vi "S19 Read.vi"(8 "error in":errorcluster, 11 "Flash File Path":path=path "D:/Gex 2 Flash Tool/SW_1_9_7_CT_0_4_2.s19") -> (0 "error out":errorcluster, 3 "Messages":T1[](array[typedef]) {"address" format="%x"; "Byte Array" format="%.0x"})   [LabVIEW 2018]
uses:
  type defs/s messages.ctl
panel:
  in  "message length (nibbles)":i32=512
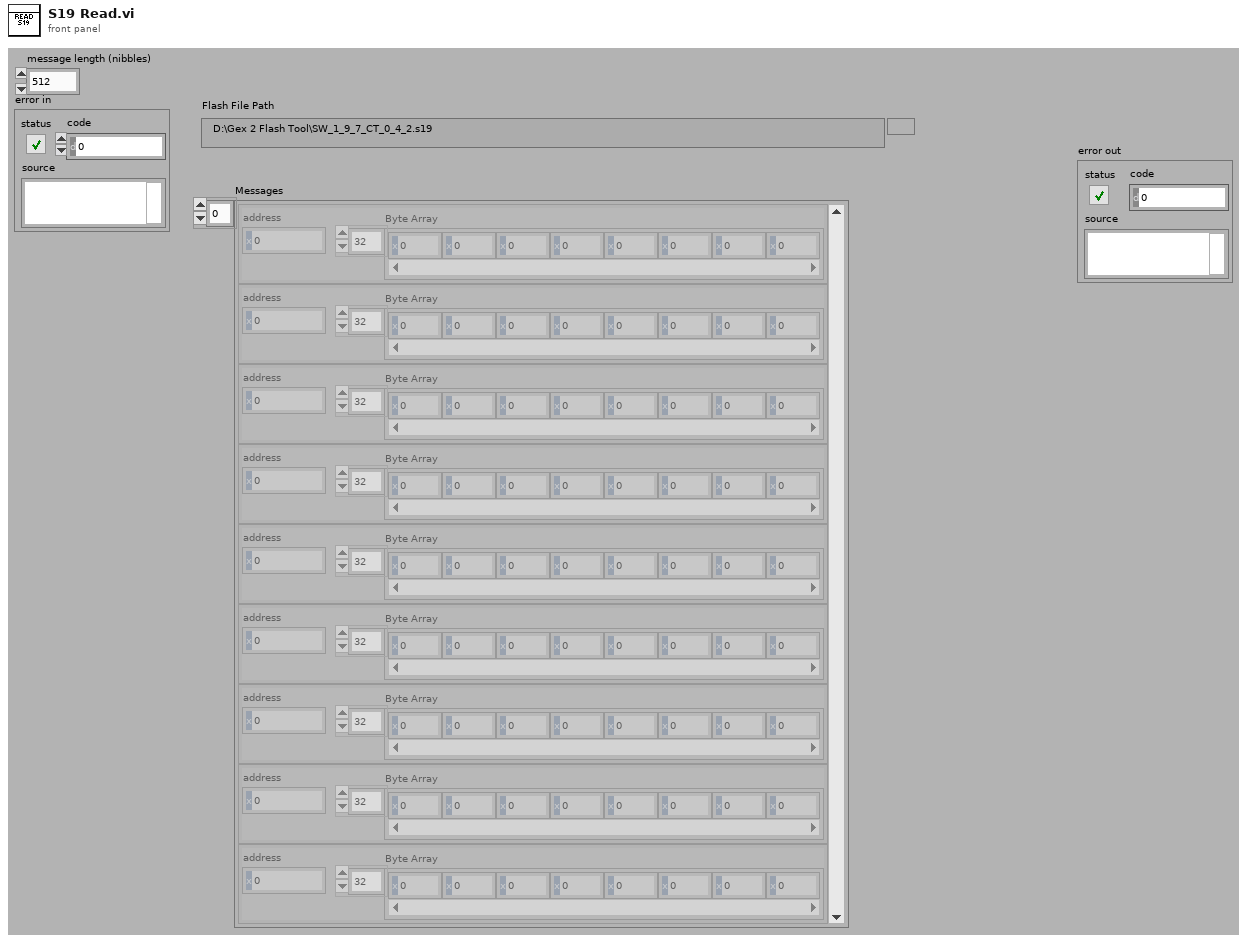
[diagram p1: front panel]
types:
  T1 = typedef "s messages.ctl" = cluster{"address":u32, "Byte Array":u8[]}
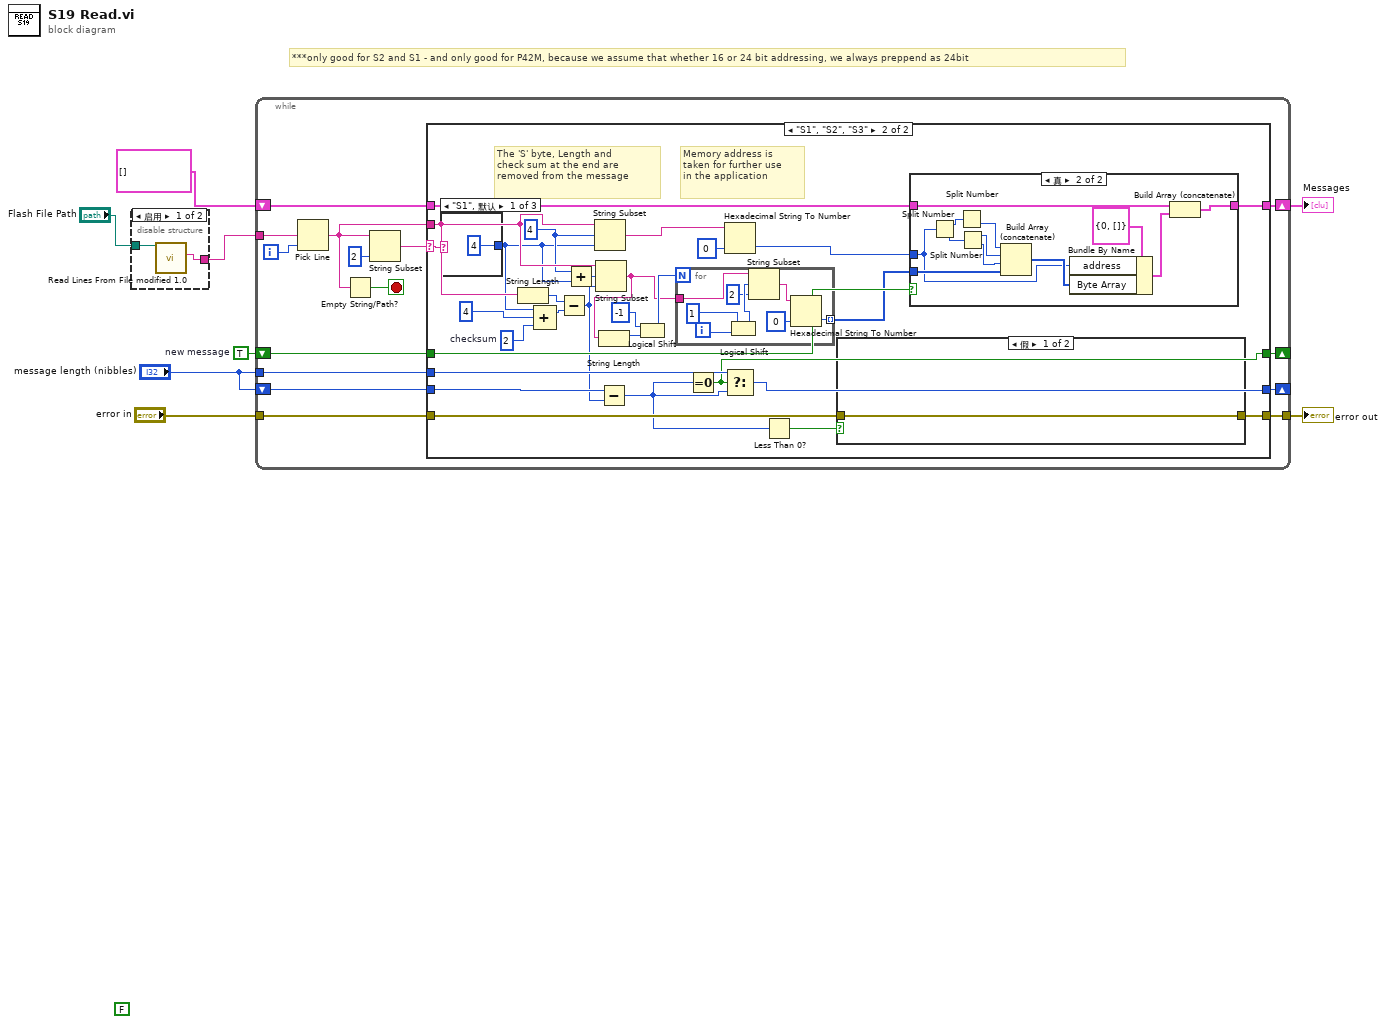
[diagram p0: block diagram]
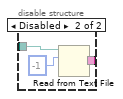
[diagram p2: hidden frame]
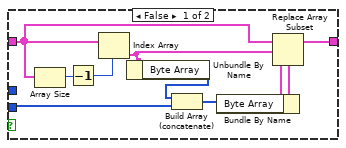
[diagram p4: hidden frame]
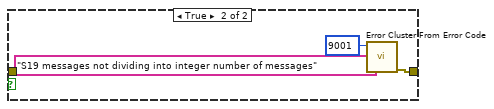
[diagram p5: hidden frame]
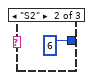
[diagram p6: hidden frame]
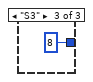
[diagram p7: hidden frame]
diagram:
  w5 = TRUE  # new message
  (unwired) FALSE
  # "***only good for S2 and S1 - and only good for P42M, because we assume that whether 16 or 24 bit addressing, we always preppend as 24bit"
  n1 = disable-structure shown="启用" {
    disable-tunnel: "Flash File Path" -> [w10 w13]
    disable-tunnel: [w9 w12] -> w1
    frame Enabled {
      n2 = call "Read Lines From File modified 1.0.vi"("file path (dialog if empty)"=w10) -> ("line string"=w9:string)  [unwired: 4 in, 4 out]
    }
    frame Disabled {
      n3 = Read from Text File(file (use dialog)=w13, count=-1 ("计数")) -> (text=w12:string)  [unwired: 2 in, 3 out]
    }
  }
  n4 = while {
    tunnel: w1 -> [w27]
    shift-right: [w21] -> w7
    shift-left: T1[] [] -> [w22]
    tunnel: "message length (nibbles)" -> [w20]
    shift-right: [w18] -> _
    shift-left: "message length (nibbles)" -> [w19]
    shift-right: [w16] -> _
    shift-left: w5 -> [w17]
    tunnel: "error in" -> [w15]
    tunnel: [w14] -> w3
    i -> [w26]
    stop <- w28 stop-if-true
    n5 = Pick Line(multi-line string=w27, line index=w26) -> (output string=w23:string)  [unwired: 1 in]
    n6 = Empty String/Path?(string/path=w23) -> (empty?=w28:bool)
    n7 = String Subset(string=w23, length (rest)=2 ("length (rest)")) -> (substring=w24:string)  [unwired: 1 in]
    n8 = case shown="\"S1\", \"S2\", \"S3\"" w24 {
      selector: w24 -> [_ w57]
      tunnel: w23 -> [_ w60]
      tunnel: w22 -> [w32 w59]
      tunnel: [w32 w58] -> w21
      tunnel: w20 -> [_ w50]
      tunnel: w19 -> [w31 w45]
      tunnel: [w31 w49] -> w18
      tunnel: w17 -> [w30 w44]
      tunnel: [w30 w43] -> w16
      tunnel: w15 -> [w29 w47]
      tunnel: [w29 w48] -> w14
      frame "False", Default {
        # "Delete out the non data S records"
      }
      frame "S1", "S2", "S3" {
        w52 = 2  # checksum
        w56 = 4 ("offset (0)")
        # "Memory address is\ntaken for further use\nin the application"
        # "The 'S' byte, Length and\ncheck sum at the end are\nremoved from the message"
        n9 = case shown="\"S1\", 默认" w57 {
          tunnel: [4 ("offset (0)") 6 ("offset (0)") 8 ("offset (0)")] -> w53
          frame "S1", Default {
          }
          frame "S2" {
          }
          frame "S3" {
          }
        }
        n10 = String Length(string=w60) -> (length=w61:i32)
        n11 = Compound Arithmetic op=ADD(w53, 4 ("value"), w52) -> (w54:i32)
        n12 = Subtract(x=w61, y=w54) -> (x-y=w38:i32)
        n13 = Add(x=w56, y=w53) -> (x+y=w55:i32)
        n14 = String Subset(string=w60, offset (0)=w56, length (rest)=w53) -> (substring=w40:string)
        n15 = String Subset(string=w60, offset (0)=w55, length (rest)=w38) -> (substring=w34:string)
        n16 = String Length(string=w34) -> (length=w36:i32)
        n17 = Subtract(x=w45, y=w38) -> (x-y=w42:i32)
        n18 = Logical Shift(y=-1 ("x"), x=w36) -> (x << y=w37:i32)
        n19 = for {
          N: w37 -> [_]
          tunnel: w34 -> [w65]
          tunnel: [w66] -> w33 mode=indexing
          i -> [w68]
          n20 = Logical Shift(y=i16 1, x=w68) -> (x << y=w63:i32)
          n21 = String Subset(string=w65, offset (0)=w63, length (rest)=2 ("length (rest)")) -> (substring=w64:string)
          n22 = Hexadecimal String To Number(string=w64, default (0uL)=u8 0 ("default (0 U32)")) -> (number=w66:u8)  [unwired: 1 in, 1 out]
        }
        n23 = Equal To 0?(x=w42) -> (x = 0?=w43:bool)
        n24 = Hexadecimal String To Number(string=w40, default (0uL)=u32 0 ("default (0 U32)")) -> (number=w39:u32)  [unwired: 1 in, 1 out]
        n25 = Select(t=w50, s=w43, f=w42) -> (s? t:f=w49:i32)
        n26 = Less Than 0?(x=w42) -> (x < 0?=w46:bool)
        n27 = case shown="假" w46 {
          tunnel: [w91 w95] -> w48
          tunnel: w47 -> [w91 w94]
          frame False {
          }
          frame True {
            n28 = call <vilib>:"Error Cluster From Error Code.vi"("error in (no error)"=w94, "error message (\"\")"="S19 messages not dividing into integer number of messages" ("error message (\"\")"), "error code (0)"=9001) -> ("error out"=w95:errorcluster)  [unwired: 6 in]
          }
        }
        n29 = case shown="真" w44 {
          tunnel: w59 -> [w77 w89]
          tunnel: [w76 w88] -> w58
          tunnel: w33 -> [w70 w86]
          tunnel: w39 -> [_ w84]
          frame False {
            n30 = Array Size(array=w77) -> (size(s)=w78:i32)
            n31 = Decrement(x=w78) -> (x-1=w73:i32)
            n32 = Index Array(array=w77, index=w73) -> (element=w75:T1)
            n33 = Unbundle By Name(w75) -> ("Byte Array"=w71:u8[])
            n34 = Build Array (concatenate)(w71, w70) -> (w72:u8[])
            n35 = Bundle By Name(cluster=w75, "Byte Array"=w72) -> (w74:T1)
            n36 = Replace Array Subset(array=w77, new element=w74, index=w73) -> (w76:T1[])
          }
          frame True {
            n37 = Split Number(x=w84) -> (hi(x)=w83:u16, lo(x)=w82:u16)
            n38 = Split Number(x=w83) -> (lo(x)=w81:u8)  [unwired: 1 out]
            n39 = Split Number(x=w82) -> (hi(x)=w79:u8, lo(x)=w80:u8)
            n40 = Build Array (concatenate)(w81, w79, w80, w86) -> (w85:u8[])
            n41 = Bundle By Name(cluster=T1 {"address"=0, "Byte Array"=[]}, "address"=w84, "Byte Array"=w85) -> (w87:T1)
            n42 = Build Array (concatenate)(w89, w87) -> (w88:T1[])
          }
        }
      }
    }
  }
  "Messages" <- w7
  "error out" <- w3
